vi "DSF.Shared.Configuration.Initialize.vi"(8 "error in (no error)":errorcluster, 9 "custom parameters":variant, 10 "name":string, 11 "Configuration in":refnum<class "DSF.Shared.Configuration.lvclass">) -> (0 "error out":errorcluster, 3 "Configuration out":refnum<class "DSF.Shared.Configuration.lvclass">)   [LabVIEW 2017, in "DSF.Shared.lvlib" / "DSF.Shared.Configuration.lvclass"]
uses:
  DSF.Shared.Configuration.lvclass
  DSF.Shared.Configuration.lvclass/DSF.Shared.Configuration.ctl
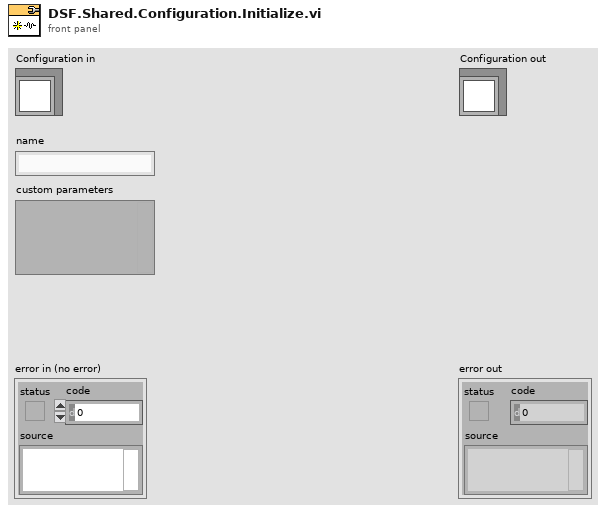
[diagram p1: front panel]
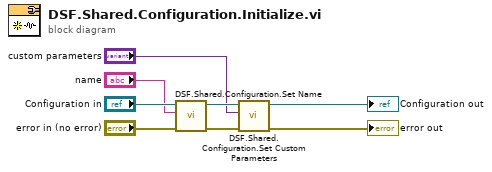
[diagram p0: block diagram]
diagram:
  n1 = call "DSF.Shared.Configuration.Set Name.vi"("name"="name", "Configuration in"="Configuration in") -> ("Configuration out"=w5:refnum<class "DSF.Shared.Configuration.lvclass">)  [unwired: 9 in]
  n2 = call "DSF.Shared.Configuration.Set Custom Parameters.vi"("custom parameters"="custom parameters", "Configuration in"=w5) -> ("Configuration out"=→"Configuration out":refnum<class "DSF.Shared.Configuration.lvclass">)  [unwired: 9 in]
  "error out" <- "error in (no error)"
